vi "FdxErrorHandler.vi"(8 "error in":errorcluster, 9 "Custom Message":string, 11 "AIM Error":i32) -> (0 "error out":errorcluster)   [LabVIEW 2020, in "AIM664LV.lvlib"]
uses:
  AIM664LV.lvlib
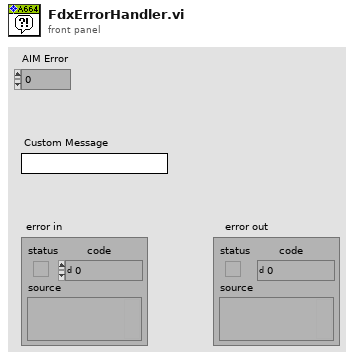
[diagram p1: front panel]
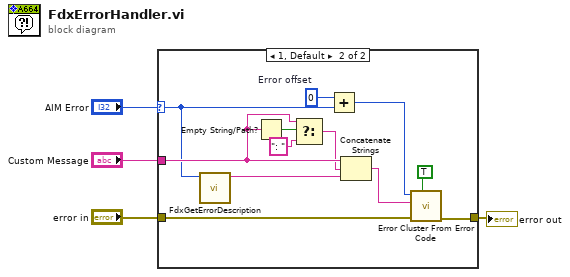
[diagram p0: block diagram]
diagram:
  n1 = case shown="1, Default" "AIM Error" {
    selector: "AIM Error" -> [_ w6]
    tunnel: "error in" -> [w5 w17]
    tunnel: [w5 w16] -> w3
    tunnel: "Custom Message" -> [_ w9]
    frame 0 {
    }
    frame 1, Default {
      w14 = 0  # Error offset
      n2 = call "FdxGetErrorDescription.vi"("fdx_error_code"=w6) -> ("string description"=w12:string)  [unwired: 9 in, 1 out]
      n3 = Empty String/Path?(string/path=w9) -> (empty?=w10:bool)
      n4 = Select(t=w9, s=w10, f=": " ("string")) -> (s? t:f=w7:string)
      n5 = Add(x=w14, y=w6) -> (x+y=w13:i32)
      n6 = Concatenate Strings(w9, w7, w12) -> (w11:string)
      n7 = call <vilib>:"Error Cluster From Error Code.vi"("show call chain? (False)"=TRUE, "error in (no error)"=w17, "error message (\"\")"=w11, "error code (0)"=w13) -> ("error out"=w16:errorcluster)  [unwired: 5 in]
    }
  }
  "error out" <- w3
